vi "Print PDF.vi"(6 "Timeout ms":i32=10000, 8 "error in (no error)":errorcluster, 9 "PDF File Path":path, 10 "printSettings":refnum<k24>, 11 "WebView2 Control in":refnum<class "WebView2 Control.lvclass">) -> (0 "error out":errorcluster, 2 "Timeout":bool, 3 "WebView2 Control out":refnum<class "WebView2 Control.lvclass">)   [LabVIEW 2020, in "WebView2.lvlib" / "WebView2 Control.lvclass"]
uses:
  WebView2 Control.lvclass
  E:/Labview/LV 2020/Libs/WebView2/LV-WebView2/Source/Libs/Microsoft.Web.WebView2.Core.dll
  Libs/Microsoft.Web.WebView2.Core.dll
  WebView2 Control.lvclass/WebView2 Control.ctl
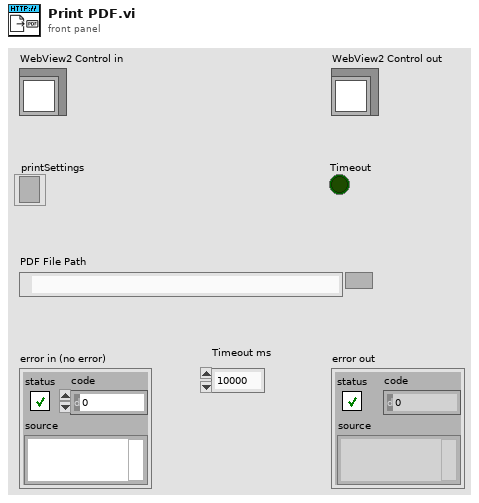
[diagram p1: front panel]
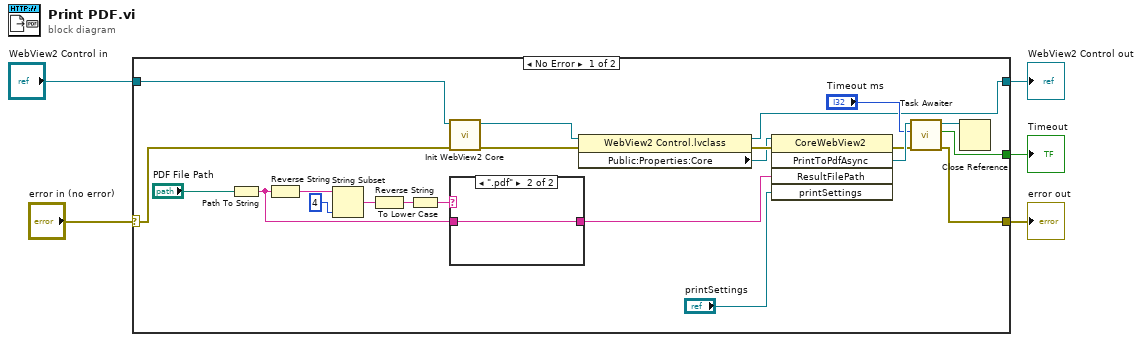
[diagram p0: block diagram]
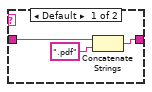
[diagram p2: hidden frame]
diagram:
  n1 = case shown="No Error" "error in (no error)" {
    selector: "error in (no error)" -> [w18 w32]
    tunnel: [w11 w32] -> w2
    tunnel: [w12 _] -> w1
    tunnel: "WebView2 Control in" -> [w19 w33]
    tunnel: [w7 w33] -> w3
    frame No Error {
      n2 = Path To String(path="PDF File Path") -> (string=w21:string)
      n3 = Reverse String(1:w21) -> (0:w27:string)
      n4 = String Subset(string=w27, length (rest)=4 ("length (rest)")) -> (substring=w25:string)  [unwired: 1 in]
      n5 = Reverse String(1:w25) -> (0:w24:string)
      n6 = To Lower Case(string=w24) -> (all lower case string=w23:string)
      n7 = call "Init WebView2 Core.vi"("error in (no error)"=w18, "WebView2"=w19) -> ("error out"=w17:errorcluster, "WebView2.lvlib:WebView2 Control.lvclass"=w8:refnum<class "WebView2 Control.lvclass">)  [unwired: 8 in]
      n8 = case shown="\".pdf\"" w23 {
        tunnel: [w28 w31] -> w22
        tunnel: w21 -> [w30 w31]
        frame Default {
          n9 = Concatenate Strings(w30, ".pdf" ("string")) -> (w28:string)
        }
        frame ".pdf" {
        }
      }
      n10 = property class="WebView2 Control.lvclass"(reference=w8, error in=w17) -> (reference out=w7:refnum<class "WebView2 Control.lvclass">, error out=w9:errorcluster, "Public:Properties:Core"=w6:refnum<k24>)
      n11 = invoke class="CoreWebView2" method="PrintToPdfAsync"(reference=w6, error in=w9, "ResultFilePath"=w22, "printSettings"="printSettings") -> (error out=w10:errorcluster, "PrintToPdfAsync"=w15:refnum<k24>)  [unwired: 1 in, 3 out]
      n12 = call "Task Awaiter.vi"("error in (no error)"=w10, "Timeout"="Timeout ms", "Task"=w15) -> ("error out"=w11:errorcluster, "Timeout"=w12:bool, "Task"=w14:refnum<k24>)  [unwired: 6 in]
      n13 = Close Reference(reference=w14) -> ()  [unwired: 1 in, 1 out]
    }
    frame Error {
    }
  }
  "error out" <- w2
  "WebView2 Control out" <- w3
  "Timeout" <- w1
